vi "EminemCmdAlign.vi"(8 "error in (no error)":errorcluster, 11 "box align":bool) -> (0 "error out":errorcluster)   [LabVIEW 2023]
uses:
  <vilib>/Rock Robotics/WPI/ThirdParty/JAS_Junk/TrajLib/Trajectory_Library.lvlib
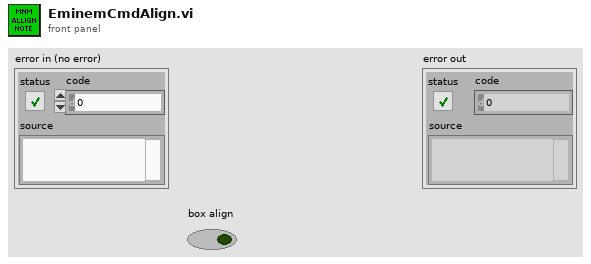
[diagram p1: front panel]
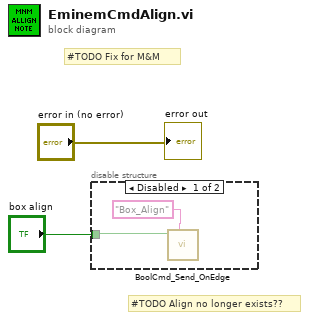
[diagram p0: block diagram]
diagram:
  # "#TODO Fix for M&M"
  # "#TODO Align no longer exists??"
  n1 = disable-structure shown="Disabled" {
    disable-tunnel: "box align" -> [w3 _]
    frame Disabled {
      n2 = call <vilib>:"BoolCmd_Send_OnEdge.vi"("Command Name"="Box_Align", "Value"=w3) -> ()  [unwired: 9 in, 1 out]
    }
    frame Enabled {
    }
  }
  "error out" <- "error in (no error)"
